vi "Test Report Contain TestCase Classname.vi"(8 "error in (no error)":errorcluster, 11 "XML Report Test in":refnum<class "XML Report Test.lvclass">) -> (0 "error out":errorcluster, 3 "XML Report Test out":refnum<class "XML Report Test.lvclass">)   [LabVIEW 2020, in "XML Report Test.lvclass"]
uses:
  XML Report Test.lvclass
  source/Plugins/XML Report/XML Report.lvclass
  XML Report Test.lvclass/XML Report Test.ctl
panel:
  out "Report Content":string
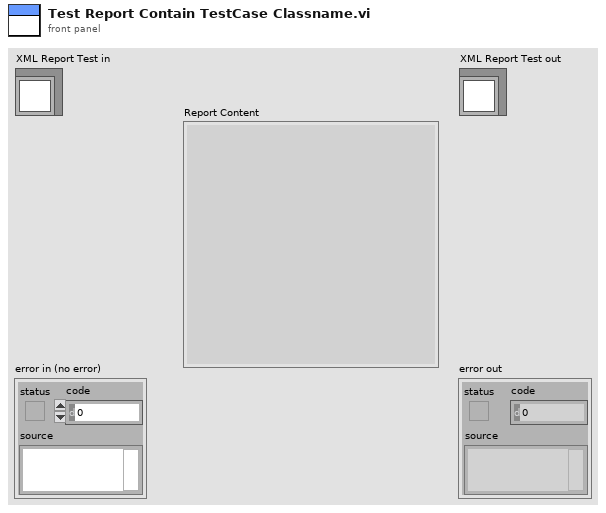
[diagram p1: front panel]
types:
  T1 = typedef "Result.lvlib/Result.ctl" = cluster{"Name":string, "Message":string, "Description":string, "Status":T2, "Result Type":T3, "Execution Time":dbl}
  T2 = typedef "Result.lvlib/Status.ctl" = enum16{"", "Passed", "Failed", "Error", "Skipped", "Setup Error", "Broken", "Teardown Error"}
  T3 = typedef "Result.lvlib/Type.ctl" = enum16{"Test Case", "Test Suite", "Test Run", "Pass", "Fail", "Skip", "Pass if", "Fail if", "Pass if Error", "Fail if Error", "Pass if Equal", "Fail if Equal"}
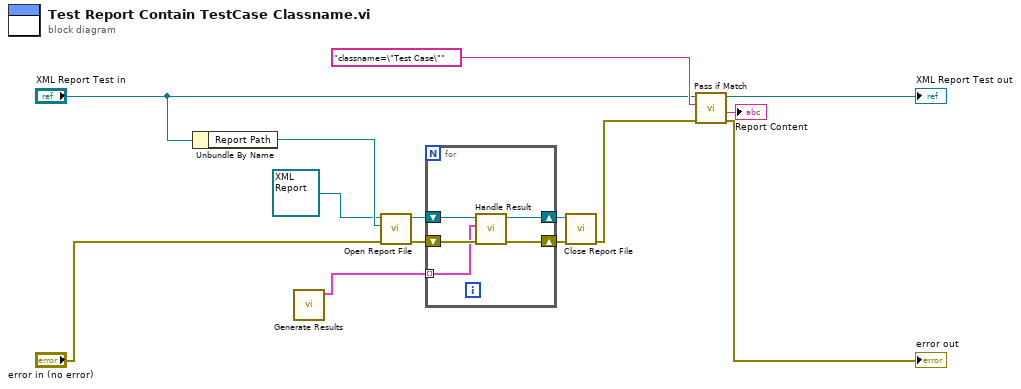
[diagram p0: block diagram]
diagram:
  n1 = Unbundle By Name("XML Report Test in") -> ("Report Path"=w9:path)
  n2 = call "Generate Results.vi"() -> ("Data"=w3:T1[])  [unwired: 10 in, 1 out]
  n3 = call-dynamic "Open Report File.vi"("error in (no error)"="error in (no error)", "Report Path"=w9, "XML Report In"=refnum<class "XML Report.lvclass"> refnum) -> ("error out"=w14:errorcluster, "XML Report Out"=w5:refnum<class "XML Report.lvclass">)  [unwired: 7 in]
  n4 = for {
    shift-right: [w18] -> w6
    shift-left: w14 -> [w19]
    shift-right: [w16] -> w4
    shift-left: w5 -> [w17]
    tunnel: w3 -> [w15] mode=indexing
    n5 = call-dynamic "Handle Result.vi"("error in (no error)"=w19, "Result"=w15, "XML Report In"=w17) -> ("error out"=w18:errorcluster, "XML Report Out"=w16:refnum<class "XML Report.lvclass">)  [unwired: 7 in]
  }
  n6 = call-dynamic "Close Report File.vi"("error in (no error)"=w6, "XML Report In"=w4) -> ("error out"=w11:errorcluster)  [unwired: 8 in, 1 out]
  n7 = call "Pass if Match.vi"("error in (no error)"=w11, "regular expression"="classname=\"Test Case\"", "XML Report Test in"="XML Report Test in") -> ("error out"=→"error out":errorcluster, "Report Content"=→"Report Content":string, "XML Report Test out"=→"XML Report Test out":refnum<class "XML Report Test.lvclass">)  [unwired: 6 in]
